vi "LogTest.vi"() -> ()   [LabVIEW 2014]
uses:
  <vilib>/Analysis/NI_AALBase.lvlib
  <vilib>/Analysis/1siggen.llb/Ramp Pattern by Samples.vi
panel:
  out "XY Graph":cluster{"X":dbl, "Y":dbl}[](graph)
  out "Waveform Graph":dbl[][](graph)
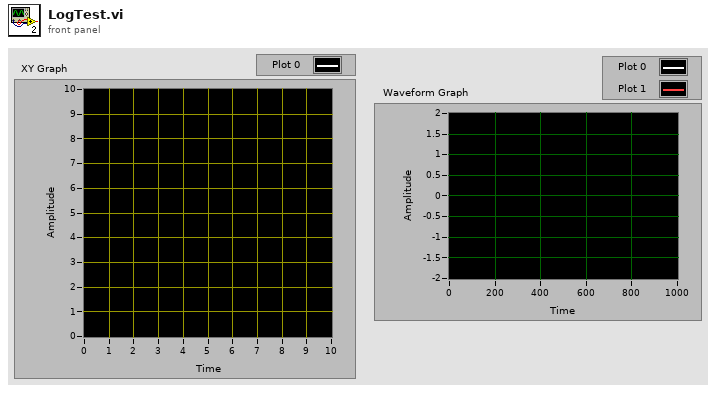
[diagram p1: front panel]
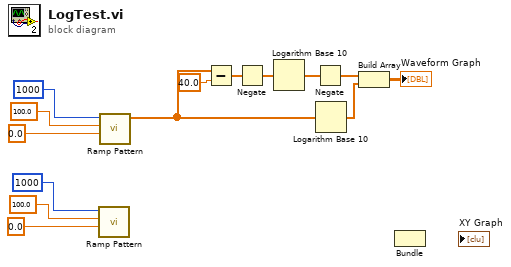
[diagram p0: block diagram]
diagram:
  n1 = call-poly <vilib>:"Ramp Pattern.vi"("start"=0.0, "end"=100.0, "samples"=1000) -> ()  [unwired: 7 in, 2 out]
  n2 = call-poly <vilib>:"Ramp Pattern.vi"("start"=0.0, "end"=100.0, "samples"=1000) -> ("Ramp Pattern"=w11:dbl[])  [unwired: 7 in, 1 out]
  n3 = Subtract(x=w11, y=40.0) -> (x-y=w10:dbl[])
  n4 = Negate(x=w10) -> (-x=w4:dbl[])
  n5 = Logarithm Base 10(1:w4) -> (0:w8:dbl[])
  n6 = Negate(x=w8) -> (-x=w5:dbl[])
  n7 = Logarithm Base 10(1:w11) -> (0:w7:dbl[])
  n8 = Build Array(w5, w7) -> (→"Waveform Graph":dbl[][])
  n9 = Bundle() -> ()  [unwired: 3 in, 1 out]
